vi "SetColor.vi"(8 "error in (no error)":errorcluster, 10 "Color":u32(colorbox), 11 "ColorRGB in":refnum<class "ColorCMYK.lvclass">) -> (0 "error out":errorcluster, 3 "ColorRGB out":refnum<class "ColorCMYK.lvclass">)   [LabVIEW 2021, in "Picture2D.lvlib" / "ColorCMYK.lvclass"]
uses:
  ColorCMYK.lvclass
  Color/Color.lvclass
  ColorCMYK.lvclass/ColorCMYK.ctl
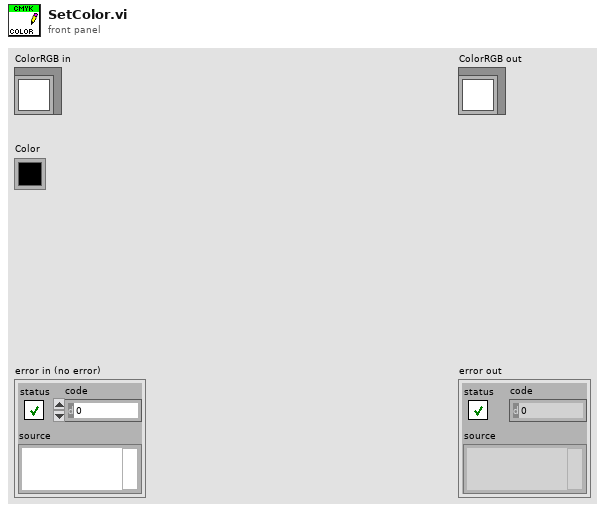
[diagram p1: front panel]
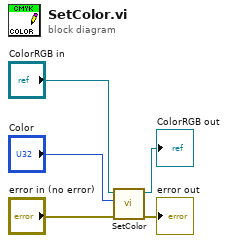
[diagram p0: block diagram]
diagram:
  n1 = call-parent "SetColor.vi"("error in (no error)"="error in (no error)", "Color"="Color", "Color in"="ColorRGB in") -> ("error out"=→"error out":errorcluster, "Color out"=→"ColorRGB out":refnum<class "ColorCMYK.lvclass">)  [unwired: 7 in]
